vi "Log Message.vi"(7 "Time Stamp":timestamp, 8 "error in (no error)":errorcluster, 9 "Message":refnum<class "Message.lvclass">, 10 "Receiving Actor":refnum<class "Message Enqueuer.lvclass">, 11 "Actor Monitor in":refnum<class "Actor Monitor.lvclass">) -> (0 "error out":errorcluster, 3 "Actor Monitor out":refnum<class "Actor Monitor.lvclass">)   [LabVIEW 2017, in "MGI-Monitored Actor Core.lvlib" / "Actor Monitor.lvclass"]
uses:
  Actor Monitor.lvclass
  <vilib>/ActorFramework/Message/Message.lvclass
  <vilib>/ActorFramework/Message Enqueuer/Message Enqueuer.lvclass
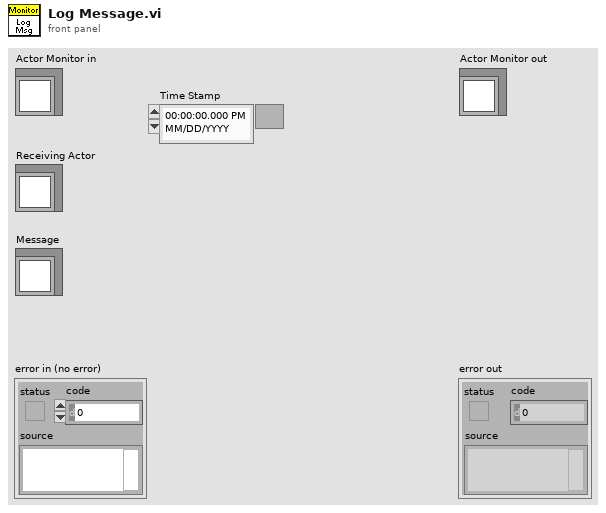
[diagram p1: front panel]
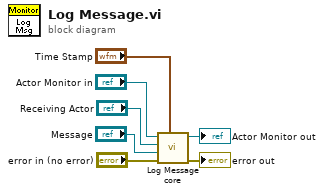
[diagram p0: block diagram]
diagram:
  n1 = call-dynamic "Log Message core.vi"("Time Stamp"="Time Stamp", "error in (no error)"="error in (no error)", "Message"="Message", "Receiving Actor"="Receiving Actor", "Actor Monitor in"="Actor Monitor in") -> ("error out"=→"error out":errorcluster, "Actor Monitor out"=→"Actor Monitor out":refnum<class "Actor Monitor.lvclass">)  [unwired: 5 in]
